vi "Write Error Status (Single).vi"(8 "error in":errorcluster, 9 "Channel Index":i32=1, 10 "Error":errorcluster, 11 "Cycler in":refnum<class "Cycler.lvclass">) -> (0 "error out":errorcluster, 3 "Cycler out":refnum<class "Cycler.lvclass">)   [LabVIEW 2023, in "Cycler.lvclass"]
uses:
  Cycler.lvclass
  Cycler.lvclass/Cycler.ctl
  <vilib>/ADAS Replay HIL/Channels/Tag Wrapper/Polymorphic/Write Channel (I32).vi
  <vilib>/ADAS Replay HIL/Channels/Tag Wrapper/Polymorphic/Write Channel (I32).vi/cccb8e89-591f-4bb4-9d4e-ae06ba1f5498.vi
  <vilib>/ADAS Replay HIL/Channels/Tag Wrapper/Polymorphic/Write Channel (I32).vi/cccb8e89-591f-4bb4-9d4e-ae06ba1f5498.vi/4bc1c15b-36ab-481f-b8dd-c64075ce723a.vi
  <vilib>/ADAS Replay HIL/Channels/Tag Wrapper/Polymorphic/Write Channel (I32).vi/cccb8e89-591f-4bb4-9d4e-ae06ba1f5498.vi/d83cb72b-7713-41fc-a3d1-682de79cf574.vi
  <vilib>/ADAS Replay HIL/Channels/Tag Wrapper/Tag Wrapper.lvlib
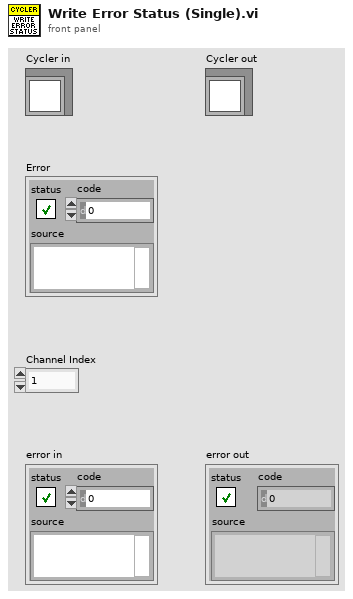
[diagram p1: front panel]
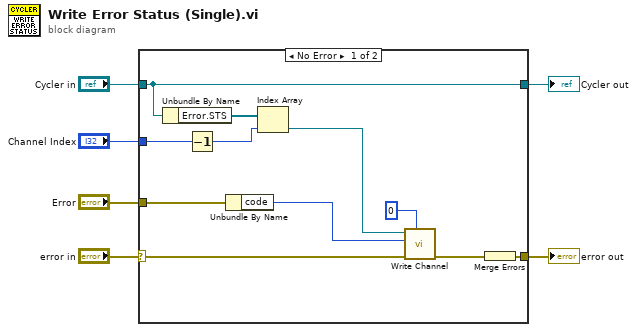
[diagram p0: block diagram]
diagram:
  n1 = case shown="No Error" "error in" {
    selector: "error in" -> [w15 w18]
    tunnel: [w12 w18] -> w5
    tunnel: [w17 w19] -> w3
    tunnel: "Cycler in" -> [w17 w19]
    tunnel: "Error" -> [w13 _]
    tunnel: "Channel Index" -> [w10 _]
    frame No Error {
      n2 = Unbundle By Name(w17) -> ("Error.STS"=w14:refnum<k21>[])
      n3 = Decrement(x=w10) -> (x-1=w9:i32)
      n4 = Unbundle By Name(w13) -> ("code"=w8:i32)
      n5 = Index Array(array=w14, index=w9) -> (element=w11:refnum<k21>)
      n6 = call-poly <vilib>:"Write Channel.vi"("Timeout (ms)"=0, "error in"=w15, "Value to Write"=w8, "ADAS HIL Channel in"=w11) -> ("error out"=w16:errorcluster)  [unwired: 5 in, 2 out]
      n7 = Merge Errors(w16) -> (w12:errorcluster)
    }
    frame Error {
    }
  }
  "error out" <- w5
  "Cycler out" <- w3
